vi "Save Meter Data.vi"(11 "VISA resource name":refnum<visa-resource-name>) -> ()   [LabVIEW 2013]
uses:
  <instrlib>/Watts Up Series/Watts Up Series.lvlib
panel:
  in  "Path":path
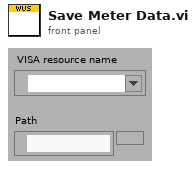
[diagram p1: front panel]
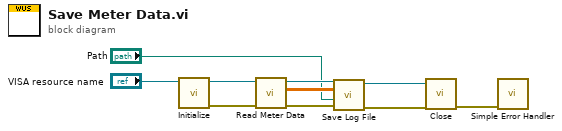
[diagram p0: block diagram]
diagram:
  n1 = call <instrlib>:"Initialize.vi"("VISA resource name"="VISA resource name") -> ("error out"=w8:errorcluster, "VISA resource name out"=w9:refnum<visa-resource-name>)  [unwired: 9 in]
  n2 = call <instrlib>:"Read Meter Data.vi"("error in (no error)"=w8, "VISA resource name"=w9) -> ("error out"=w6:errorcluster, "Logged Data"=w5:dbl[][], "VISA resource name out"=w7:refnum<visa-resource-name>)  [unwired: 7 in]
  n3 = call <instrlib>:"Save Log File.vi"("error in (no error)"=w6, "Path"="Path", "Logged Data"=w5, "VISA resource name"=w7) -> ("error out"=w2:errorcluster, "VISA resource name out"=w3:refnum<visa-resource-name>)  [unwired: 6 in]
  n4 = call <instrlib>:"Close.vi"("error in (no error)"=w2, "VISA resource name"=w3) -> ("error out"=w1:errorcluster)  [unwired: 9 in]
  n5 = call <vilib>:"Simple Error Handler.vi"("error in (no error)"=w1) -> ()  [unwired: 4 in, 5 out]
